vi "PipelineDuty.vi"(8 "error in (no error)":errorcluster, 10 "DataExchange":T1, 11 "GRMActor in":refnum<class "FlatFieldUI.lvclass">) -> (0 "error out":errorcluster, 2 "DataExchange Out":T1, 3 "GRMActor out":refnum<class "FlatFieldUI.lvclass">)   [LabVIEW 2020, in "FlatFieldUI.lvlib" / "FlatFieldUI.lvclass"]
uses:
  FlatFieldUI.lvclass
  Hardware Abstraction Layer/Component/Device/Device/DataExchange.ctl
  <vilib>/vision/Image Controls.llb/IMAQ Image.ctl
  FlatFieldUI.lvclass/FlatFieldUI.ctl
  FlatField/FlatField/FlatField Status.ctl
  Hardware Abstraction Layer/Component/GenericActor/GenericActor/GenericController.lvclass
  Interface/DataListener/DataListener.lvclass
  <vilib>/vision/NI_Vision_Development_Module.lvlib
panel:
  out "Source":string
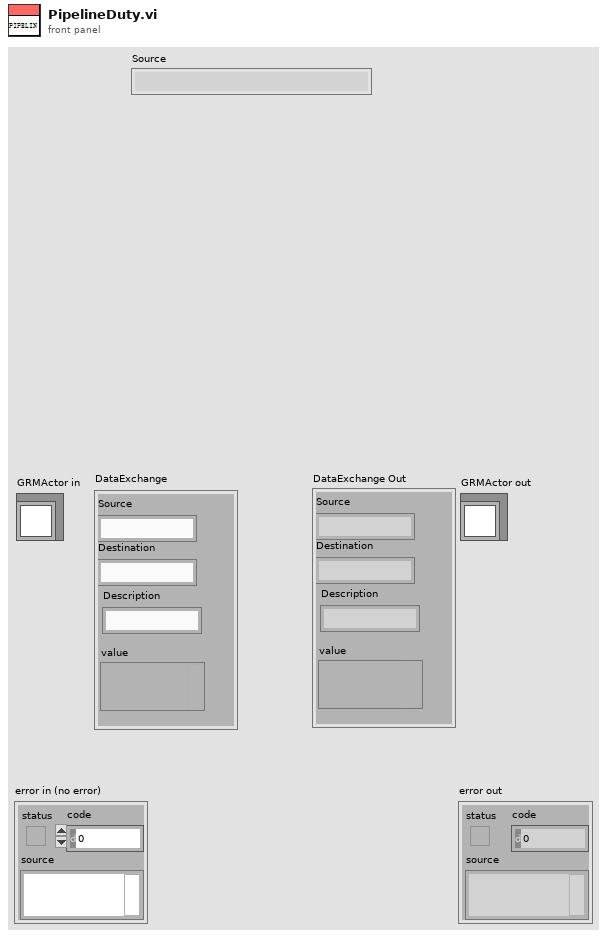
[diagram p1: front panel]
types:
  T1 = typedef "DataListener.lvclass/DataExchange.ctl" = cluster{"Source":string, "Destination":string, "Description":string, "value":variant}
  T2 = typedef "IMAQ Image.ctl" = refnum<image>
  T3 = typedef "FlatFieldUI.lvlib/FlatFieldUI.lvclass/FlatField Status.ctl" = i32
  T4 = typedef "FlatFieldUI.lvlib/FlatFieldUI.lvclass/FlatField Method.ctl" = i32
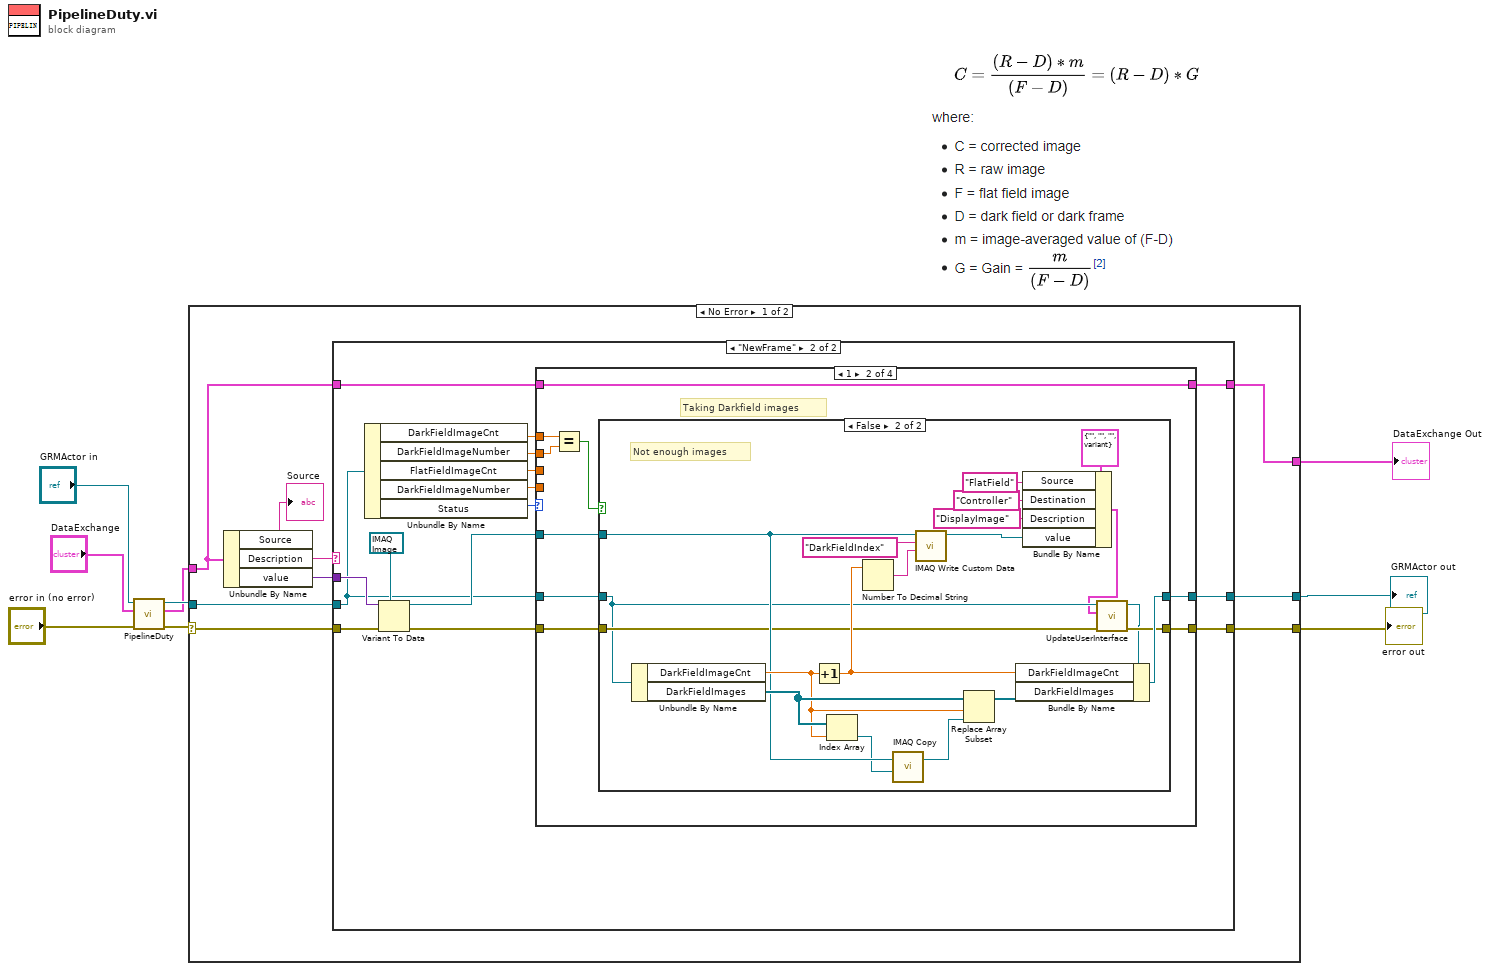
[diagram p0: block diagram]
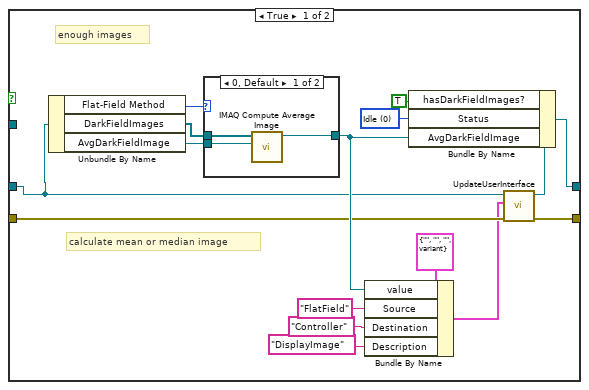
[diagram p4: hidden frame]
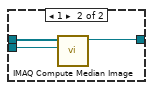
[diagram p5: hidden frame]
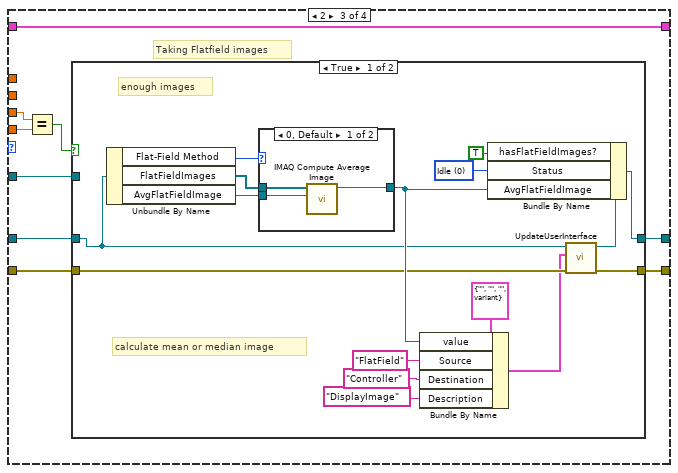
[diagram p6: hidden frame]
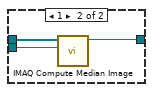
[diagram p7: hidden frame]
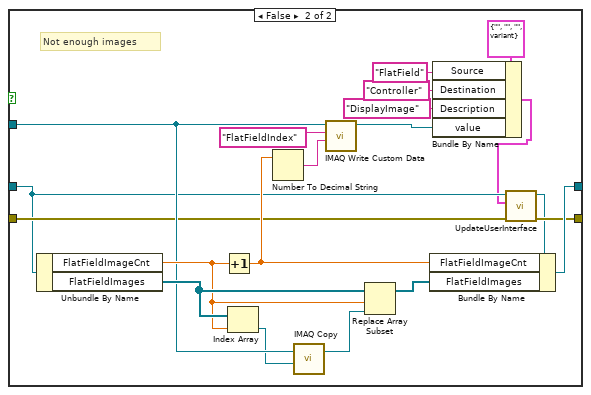
[diagram p8: hidden frame]
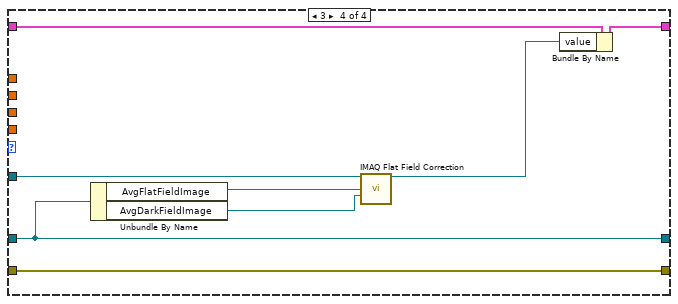
[diagram p9: hidden frame]
diagram:
  n1 = call-parent "PipelineDuty.vi"("error in (no error)"="error in (no error)", "DataExchange"="DataExchange", "GRMActor in"="GRMActor in") -> ("error out"=w6:errorcluster, "DataExchange Out"=w4:T1, "GRMActor out"=w5:refnum<class "FlatFieldUI.lvclass">)  [unwired: 6 in]
  n2 = case shown="No Error" w6 {
    selector: w6 -> [w16 w152]
    tunnel: [w17 w152] -> w3
    tunnel: w5 -> [w13 w151]
    tunnel: [w18 w151] -> w2
    tunnel: w4 -> [w12 w150]
    tunnel: [w11 w150] -> w1
    frame No Error {
      n3 = Unbundle By Name(w12) -> ("Source"=→"Source":string, "Description"=w15:string, "value"=w14:variant)
      n4 = case shown="\"NewFrame\"" w15 {
        tunnel: w14 -> [_ w35]
        tunnel: [w21 w31] -> w18
        tunnel: w13 -> [w21 w29]
        tunnel: [w20 w32] -> w17
        tunnel: w16 -> [w20 w36]
        tunnel: w12 -> [w19 w23]
        tunnel: [w19 w22] -> w11
        frame Default {
        }
        frame "NewFrame" {
          n5 = Unbundle By Name(w29) -> ("DarkFieldImageCnt"=w27:dbl, "DarkFieldImageNumber"=w26:dbl, "FlatFieldImageCnt"=w25:dbl, "DarkFieldImageNumber"=w24:dbl, "Status"=w28:T3)
          n6 = Variant To Data(error in=w36, type=T2 refnum ("New Image"), Variant=w35) -> (data=w30:T2, error out=w33:errorcluster)
          n7 = case shown="1" w28 {
            tunnel: w33 -> [w38 w48 w99 w149]
            tunnel: [w38 w47 w98 w149] -> w32
            tunnel: [w39 w46 w97 w147] -> w31
            tunnel: w30 -> [_ w44 w95 w145]
            tunnel: w29 -> [w39 w45 w96 w147]
            tunnel: w27 -> [_ w43 _ _]
            tunnel: w26 -> [_ w42 _ _]
            tunnel: w25 -> [_ _ w92 _]
            tunnel: w24 -> [_ _ w91 _]
            tunnel: w23 -> [w37 w40 w93 w148]
            tunnel: [w37 w40 w93 w146] -> w22
            frame 0, Default {
              # "idle"
            }
            frame 1 {
              # "Taking Darkfield images"
              n8 = Equal?(x=w43, y=w42) -> (x = y?=w41:bool)
              n9 = case shown="False" w41 {
                tunnel: w48 -> [w53 w75]
                tunnel: [w52 w74] -> w47
                tunnel: [w56 w82] -> w46
                tunnel: w45 -> [w50 w72]
                tunnel: w44 -> [_ w78]
                frame True {
                  w55 = T3 0 items=["Idle", "Taking DarkField Images", "Taking FlatField Image", "Doing FlatField", ""] ("Flat-Field Status")
                  # "calculate mean or median image"
                  # "enough images"
                  n10 = Unbundle By Name(w50) -> ("Flat-Field Method"=w58:T4, "DarkFieldImages"=w60:T2[], "AvgDarkFieldImage"=w59:T2)
                  n11 = case shown="0, Default" w58 {
                    tunnel: [w65 w70] -> w57
                    tunnel: w60 -> [w67 w69]
                    tunnel: w59 -> [w66 w68]
                    frame 0, Default {
                      n12 = call "IMAQ Compute Average Image"("Image Dst"=w66, "Images"=w67) -> ("Image Dst Out"=w65:T2)  [unwired: 8 in, 1 out]
                    }
                    frame 1 {
                      n13 = call "IMAQ Compute Median Image"("Image Dst"=w68, "Images"=w69) -> ("Image Dst Out"=w70:T2)  [unwired: 8 in, 1 out]
                    }
                  }
                  n14 = Bundle By Name(cluster=T1 {"Source"="", "Destination"="", "Description"="", "value"=variant} ("DataExchange"), "value"=w57, "Source"="FlatField", "Destination"="Controller", "Description"="DisplayImage") -> (w49:T1)
                  n15 = call-dynamic "UpdateUserInterface.vi"("error in (no error)"=w53, "DataExchange"=w49, "FlatFieldUI in"=w50) -> ("error out"=w52:errorcluster, "FlatFieldUI out"=w51:refnum<class "FlatFieldUI.lvclass">)  [unwired: 6 in, 1 out]
                  n16 = Bundle By Name(cluster=w51, "hasDarkFieldImages?"=TRUE, "Status"=w55, "AvgDarkFieldImage"=w57) -> (w56:refnum<class "FlatFieldUI.lvclass">)
                }
                frame False {
                  # "Not enough images"
                  n17 = Unbundle By Name(w72) -> ("DarkFieldImageCnt"=w79:dbl, "DarkFieldImages"=w80:T2[])
                  n18 = Increment(x=w79) -> (x+1=w83:dbl)
                  n19 = Index Array "Index Array"(array=w80, index=w79) -> (element=w77:T2)
                  n20 = Number To Decimal String(number=w83) -> (decimal integer string=w84:string)  [unwired: 1 in]
                  n21 = call "IMAQ Copy"("Image Dst"=w77, "Image Src"=w78) -> ("Image Dst Out"=w76:T2)  [unwired: 4 in, 1 out]
                  n22 = call "IMAQ Write Custom Data"("Custom Data In"=w84, "Key"="DarkFieldIndex", "Image"=w78) -> ("Image Out"=w86:T2)  [unwired: 7 in, 1 out]
                  n23 = Replace Array Subset "Replace Array Subset"(array=w80, new element=w76, index=w79) -> (w81:T2[])
                  n24 = Bundle By Name(cluster=T1 {"Source"="", "Destination"="", "Description"="", "value"=variant} ("DataExchange"), "Source"="FlatField", "Destination"="Controller", "Description"="DisplayImage", "value"=w86) -> (w71:T1)
                  n25 = call-dynamic "UpdateUserInterface.vi"("error in (no error)"=w75, "DataExchange"=w71, "FlatFieldUI in"=w72) -> ("error out"=w74:errorcluster, "FlatFieldUI out"=w73:refnum<class "FlatFieldUI.lvclass">)  [unwired: 6 in, 1 out]
                  n26 = Bundle By Name(cluster=w73, "DarkFieldImageCnt"=w83, "DarkFieldImages"=w81) -> (w82:refnum<class "FlatFieldUI.lvclass">)
                }
              }
            }
            frame 2 {
              # "Taking Flatfield images"
              n27 = Equal?(x=w92, y=w91) -> (x = y?=w94:bool)
              n28 = case shown="True" w94 {
                tunnel: w99 -> [w104 w126]
                tunnel: [w103 w125] -> w98
                tunnel: [w107 w133] -> w97
                tunnel: w96 -> [w101 w123]
                tunnel: w95 -> [_ w128]
                frame True {
                  w106 = T3 0 items=["Idle", "Taking DarkField Images", "Taking FlatField Image", "Doing FlatField", ""] ("Flat-Field Status")
                  # "calculate mean or median image"
                  # "enough images"
                  n29 = Unbundle By Name(w101) -> ("Flat-Field Method"=w109:T4, "FlatFieldImages"=w111:T2[], "AvgFlatFieldImage"=w110:T2)
                  n30 = case shown="0, Default" w109 {
                    tunnel: [w116 w121] -> w108
                    tunnel: w111 -> [w118 w120]
                    tunnel: w110 -> [w117 w119]
                    frame 0, Default {
                      n31 = call "IMAQ Compute Average Image"("Image Dst"=w117, "Images"=w118) -> ("Image Dst Out"=w116:T2)  [unwired: 8 in, 1 out]
                    }
                    frame 1 {
                      n32 = call "IMAQ Compute Median Image"("Image Dst"=w119, "Images"=w120) -> ("Image Dst Out"=w121:T2)  [unwired: 8 in, 1 out]
                    }
                  }
                  n33 = Bundle By Name(cluster=T1 {"Source"="", "Destination"="", "Description"="", "value"=variant} ("DataExchange"), "value"=w108, "Source"="FlatField", "Destination"="Controller", "Description"="DisplayImage") -> (w100:T1)
                  n34 = call-dynamic "UpdateUserInterface.vi"("error in (no error)"=w104, "DataExchange"=w100, "FlatFieldUI in"=w101) -> ("error out"=w103:errorcluster, "FlatFieldUI out"=w102:refnum<class "FlatFieldUI.lvclass">)  [unwired: 6 in, 1 out]
                  n35 = Bundle By Name(cluster=w102, "hasFlatFieldImages?"=TRUE, "Status"=w106, "AvgFlatFieldImage"=w108) -> (w107:refnum<class "FlatFieldUI.lvclass">)
                }
                frame False {
                  # "Not enough images"
                  n36 = Unbundle By Name(w123) -> ("FlatFieldImageCnt"=w129:dbl, "FlatFieldImages"=w131:T2[])
                  n37 = Increment(x=w129) -> (x+1=w134:dbl)
                  n38 = Index Array(array=w131, index=w129) -> (element=w127:T2)
                  n39 = Number To Decimal String(number=w134) -> (decimal integer string=w135:string)  [unwired: 1 in]
                  n40 = call "IMAQ Copy"("Image Dst"=w127, "Image Src"=w128) -> ("Image Dst Out"=w132:T2)  [unwired: 4 in, 1 out]
                  n41 = call "IMAQ Write Custom Data"("Custom Data In"=w135, "Key"="FlatFieldIndex", "Image"=w128) -> ("Image Out"=w137:T2)  [unwired: 7 in, 1 out]
                  n42 = Replace Array Subset "Replace Array Subset"(array=w131, new element=w132, index=w129) -> (w130:T2[])
                  n43 = Bundle By Name(cluster=T1 {"Source"="", "Destination"="", "Description"="", "value"=variant} ("DataExchange"), "Source"="FlatField", "Destination"="Controller", "Description"="DisplayImage", "value"=w137) -> (w122:T1)
                  n44 = call-dynamic "UpdateUserInterface.vi"("error in (no error)"=w126, "DataExchange"=w122, "FlatFieldUI in"=w123) -> ("error out"=w125:errorcluster, "FlatFieldUI out"=w124:refnum<class "FlatFieldUI.lvclass">)  [unwired: 6 in, 1 out]
                  n45 = Bundle By Name(cluster=w124, "FlatFieldImageCnt"=w134, "FlatFieldImages"=w130) -> (w133:refnum<class "FlatFieldUI.lvclass">)
                }
              }
            }
            frame 3 {
              n46 = Unbundle By Name(w147) -> ("AvgFlatFieldImage"=w144:T2, "AvgDarkFieldImage"=w143:T2)
              n47 = call "IMAQ Flat Field Correction"("Image Src"=w145, "Flat Field Image"=w144, "Dark Field Image"=w143) -> ("Corrected Image"=w142:T2)  [unwired: 10 in, 2 out]
              n48 = Bundle By Name(cluster=w148, "value"=w142) -> (w146:T1)
            }
          }
        }
      }
    }
    frame Error {
    }
  }
  "error out" <- w3
  "GRMActor out" <- w2
  "DataExchange Out" <- w1
